vi "Update UI per Reference.vi"(8 "error in (no error)":errorcluster, 11 "Analyze Results FF-Spectrum in":refnum<class "Analyze Results FF-Spectrum.lvclass">) -> (0 "error out":errorcluster, 3 "Analyze Results FF-Spectrum out":refnum<class "Analyze Results FF-Spectrum.lvclass">)   [LabVIEW 2020, in "Analyze Results FF-Spectrum.lvclass"]
uses:
  Analyze Results FF-Spectrum.lvclass
  Analyze Results FF-Spectrum.lvclass/Analyze Results FF-Spectrum.ctl
  Results Base/Analyze Results Base.lvclass
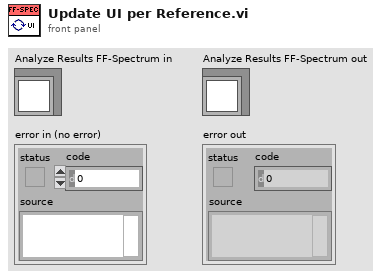
[diagram p1: front panel]
types:
  T1 = typedef "Analyze Results FF-Spectrum.lvclass/Spectral Point.ctl" = cluster{"Wavelength":dbl[unit], "Intensity":dbl}
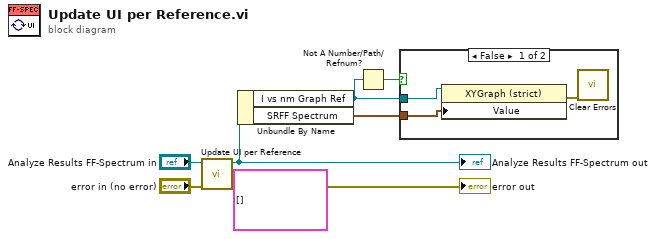
[diagram p0: block diagram]
diagram:
  (unwired) cluster{"X Values":dbl[], "mittelwerte":dbl[]}[] [] ("SRFF Graph")
  n1 = call-parent "Update UI per Reference.vi"("error in (no error)"="error in (no error)", "Analyze Results Base in"="Analyze Results FF-Spectrum in") -> ("error out"=→"error out":errorcluster, "Analyze Results Base out"=w4:refnum<class "Analyze Results FF-Spectrum.lvclass">)  [unwired: 8 in]
  "Analyze Results FF-Spectrum out" <- w4
  n2 = Unbundle By Name(w4) -> ("I vs nm Graph Ref"=w2:refnum<vi>, "SRFF Spectrum"=w1:T1[])
  n3 = Not A Number/Path/Refnum?(number/path/refnum=w2) -> (NaN/Path/Refnum?=w3:bool)
  n4 = case shown="False" w3 {
    tunnel: w2 -> [w10 _]
    tunnel: w1 -> [w8 _]
    frame False {
      n5 = property class="XYGraph (strict)"(reference=w10, "Value"=w8) -> (error out=w9:errorcluster)  [unwired: 1 in, 1 out]
      n6 = call <vilib>:"Clear Errors.vi"("error in (no error)"=w9) -> ()  [unwired: 5 in, 2 out]
    }
    frame True {
    }
  }
